vi "Write 1s_buff.vi"(8 "error in (no error)":errorcluster, 10 "1s_buff":dbl, 11 "CPC Data in":refnum<class "CPC Data.lvclass">) -> (0 "error out":errorcluster, 3 "CPC Data out":refnum<class "CPC Data.lvclass">)   [LabVIEW 2012, in "CPC Data.lvclass"]
uses:
  CPC Data.lvclass
  CPC Data.lvclass/CPC Data.ctl
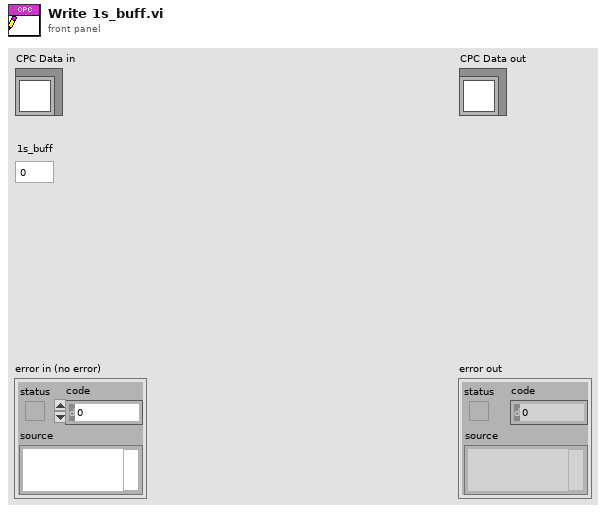
[diagram p1: front panel]
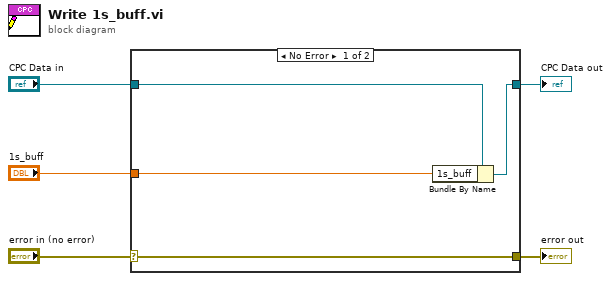
[diagram p0: block diagram]
diagram:
  n1 = case shown="No Error" "error in (no error)" {
    selector: "error in (no error)" -> [w9 w10]
    tunnel: [w9 w10] -> w4
    tunnel: [w7 w11] -> w2
    tunnel: "CPC Data in" -> [w8 w11]
    tunnel: "1s_buff" -> [w6 _]
    frame No Error {
      n2 = Bundle By Name(cluster=w8, "1s_buff"=w6) -> (w7:refnum<class "CPC Data.lvclass">)
    }
    frame Error {
    }
  }
  "error out" <- w4
  "CPC Data out" <- w2
